vi "equipoSeleccionado.vi"(8 "error in (no error)":errorcluster, 11 "Sonometro in":refnum<class "Sonometro.lvclass">) -> (0 "error out":errorcluster, 2 "equipoSeleccionado":string, 3 "Sonometro out":refnum<class "Sonometro.lvclass">)   [LabVIEW 2019, in "Sonometro.lvclass"]
uses:
  Sonometro.lvclass
  Sonometro.lvclass/Sonometro.ctl
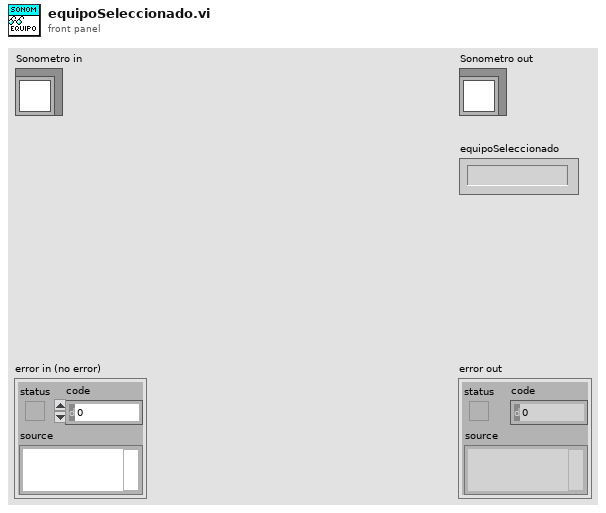
[diagram p1: front panel]
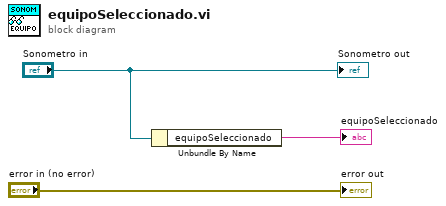
[diagram p0: block diagram]
diagram:
  n1 = Unbundle By Name("Sonometro in") -> ("equipoSeleccionado"=→"equipoSeleccionado":string)
  "error out" <- "error in (no error)"
  "Sonometro out" <- "Sonometro in"
